vi "Delete Event.vi"(8 "error in (no error)":errorcluster, 9 "DeleteAt":i32, 11 "Tosca in":refnum<class "Parameters.lvclass">) -> (0 "error out":errorcluster, 2 "Name":string, 3 "Tosca out":refnum<class "Parameters.lvclass">)   [LabVIEW 2015, in "Parameters.lvclass"]
uses:
  Parameters.lvclass
  State/State.lvclass
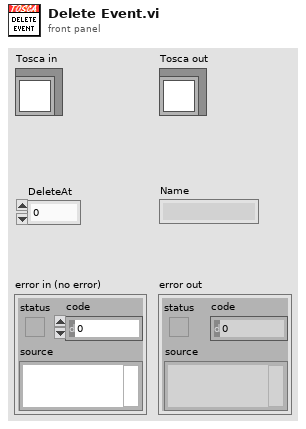
[diagram p1: front panel]
types:
  T1 = typedef "Tosca-Input Event.ctl" = cluster{"Name":string, "Criteria":T2[], "Operators":enum16{"AND", "OR"}[], "Accumulator":T4}
  T2 = typedef "Tosca-Input Criterion.ctl" = cluster{"DigInput":i32, "State":T3, "Time (ms)":i32, "Name":string}
  T3 = typedef "Logic State.ctl" = enum16{"Low", "High", "Rising", "Falling"}
  T4 = typedef "Tosca-Accumulator.ctl" = cluster{"active":bool, "N":i32, "T":dbl, "Imax":dbl, "latency":dbl}
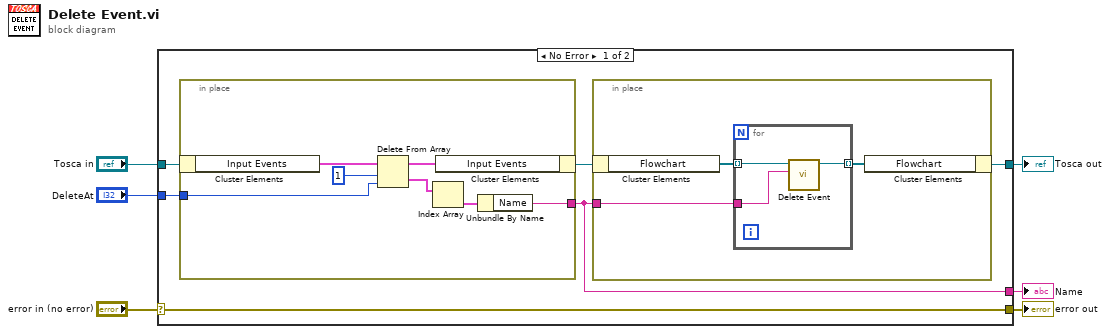
[diagram p0: block diagram]
diagram:
  n1 = case shown="No Error" "error in (no error)" {
    selector: "error in (no error)" -> [w12 w27]
    tunnel: [w12 w27] -> w5
    tunnel: [w8 w26] -> w3
    tunnel: "Tosca in" -> [w11 w26]
    tunnel: "DeleteAt" -> [w10 _]
    tunnel: [w7 _] -> w1
    frame No Error {
      n2 = in-place {
        in-place-border: w10 -> [w23]
        in-place-border: [w19] -> w7
        n3 = in-place-cluster #1(w11) -> ("Input Events"=w25:T1[])
        n4 = Delete From Array(array=w25, length=1, index=w23) -> (deleted portion=w21:T1[], array with subset deleted=w22:T1[])
        n5 = Index Array(array=w21) -> (element=w20:T1)  [unwired: 1 in]
        n6 = in-place-cluster #1("Input Events"=w22) -> (w9:refnum<class "Parameters.lvclass">)
        n7 = Unbundle By Name(w20) -> ("Name"=w19:string)
      }
      n8 = in-place {
        in-place-border: w7 -> [w14]
        n9 = in-place-cluster #2(w9) -> ("Flowchart"=w15:refnum<class "State.lvclass">[])
        n10 = for {
          tunnel: w15 -> [w18] mode=indexing
          tunnel: w14 -> [w17]
          tunnel: [w16] -> w13 mode=indexing
          n11 = call "Delete Event.vi"("Name"=w17, "State in"=w18) -> ("State out"=w16:refnum<class "State.lvclass">)  [unwired: 8 in, 1 out]
        }
        n12 = in-place-cluster #2("Flowchart"=w13) -> (w8:refnum<class "Parameters.lvclass">)
      }
    }
    frame Error {
    }
  }
  "error out" <- w5
  "Tosca out" <- w3
  "Name" <- w1
